vi "Read RFFE_w_Waveform.vi"(0 "Semiconductor Module Context":T3, 1 "USID":T1 max=15, 2 "Specific Bits Value_to_Read":cluster{"#ofBits":u8, "Bit_Location(LSB)":u8}={"#ofBits"=1, "Bit_Location(LSB)"=0} {"Bit_Location(LSB)" max=7; "#ofBits" min=1 max=8}, 5 "Pins":string[](array[string])=["CLK", "SDA"], 7 "RegisterAdd_Value_Dec":u8=28, 9 "Num_Reg_to_Read":u8, 11 "error in (no error)":errorcluster) -> (4 "Ext_Read_Reg":i32[](array[numeric]), 6 "Ext_Read_Data":u8[](array[numeric])=[31, 144, 7], 8 "Specific_Bits_Value":u8=184, 15 "error out":errorcluster)   [LabVIEW 2013]
uses:
  <vilib>/NI_TestStand_SemiconductorModule/NI_TestStand_Semiconductor_Module.lvlibp/PinMap/General/SemiconductorModuleContext.ctl
  Controls/USID.ctl
  MIPI_RFFE/Ctrls/RegReadWrite.ctl
  MIPI_RFFE/Ctrls/Configuration.ctl
  MIPI_RFFE/Ctrls/ClockDataChannels.ctl
  <instrlib>/niHSDIO/niHSDIO.llb/niHSDIO_ctl Generation Mode Values (Ring).ctl
  <vilib>/NI_TestStand_SemiconductorModule/NI_TestStand_Semiconductor_Module.lvlibp/PinMap/HSDIO/PinsToNIHSDIOSessions.vi
  <vilib>/Waveform/DWDTOps.llb/DWDT Digital Size.vi
  <instrlib>/niHSDIO/niHSDIO.llb/niHSDIO Write Named Waveform (WDT).vi
  <instrlib>/niHSDIO/niHSDIO.llb/niHSDIO Fetch Waveform (WDT).vi
  <vilib>/NI_TestStand_SemiconductorModule/NI_TestStand_Semiconductor_Module.lvlibp
panel:
  out "Converted Data":T2 {"Register" max=31 format="%.0x"; "Slave Address" max=15 format="%.0x"}
  out "Waveform Graph":digitalwaveform(graph)
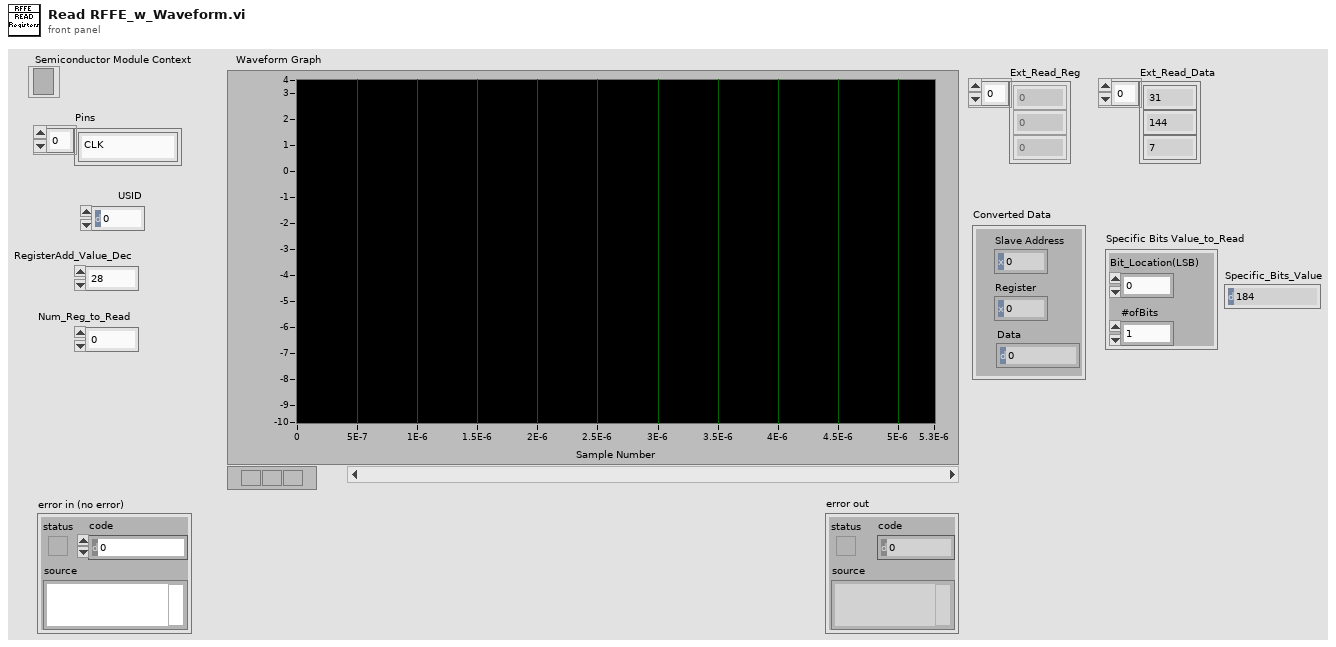
[diagram p1: front panel]
types:
  T1 = typedef "USID.ctl" = u8
  T2 = cluster{"Slave Address":u8, "Register":u8, "Data":u8}
  T3 = typedef "NI_TestStand_Semiconductor_Module.lvlibp/SemiconductorModuleContext.ctl" = refnum<k7>
  T4 = typedef "Configuration.ctl" = cluster{"Samples to Allocate":i32, "Oversample Factor":u8, "Clock Channel":T5, "Data Channel":T5}
  T5 = typedef "ClockDataChannels.ctl" = enum16{"0", "1"}
  T6 = typedef "RegReadWrite.ctl" = cluster{"Slave Address":u8, "Register":u8, "Data":u8, "SetID_Pin_State":enum16{"0", "1", "Z"}}
  T7 = typedef "niHSDIO_ctl Generation Mode Values (Ring).ctl" = i32
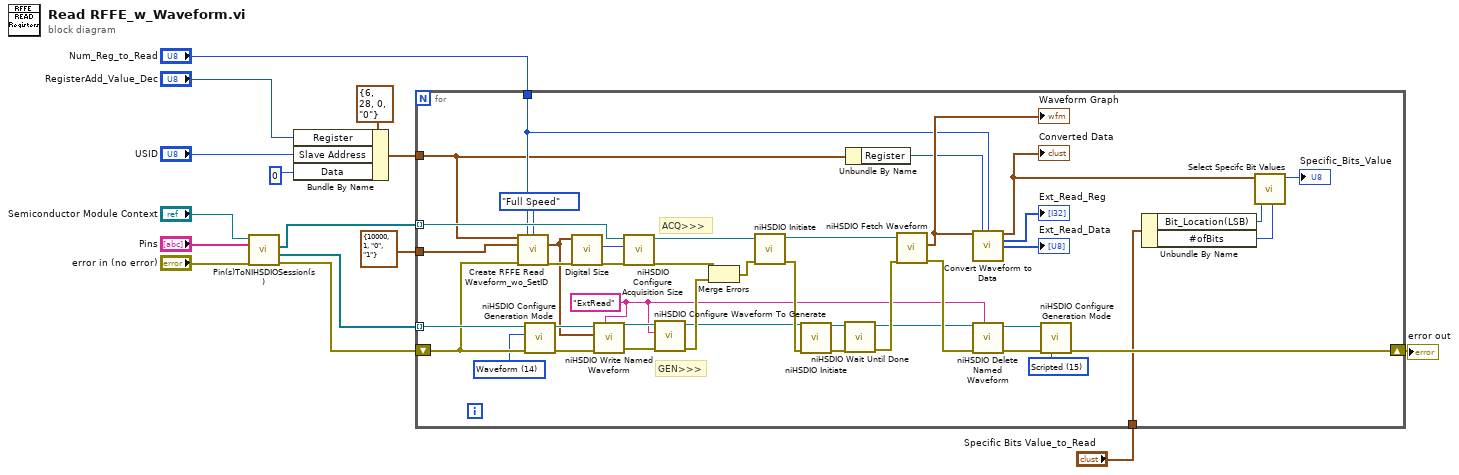
[diagram p0: block diagram]
diagram:
  n1 = call-poly <vilib>:"Pin(s)ToNIHSDIOSession(s).vi"("error in (no error)"="error in (no error)", "Pins"="Pins", "Semiconductor Module Context"="Semiconductor Module Context") -> ("error out"=w13:errorcluster, "Generation Sessions"=w14:refnum<k15>[], "Acquisition Sessions"=w15:refnum<k15>[])  [unwired: 3 in, 3 out]
  n2 = Bundle By Name(cluster=T6 {"Slave Address"=6, "Register"=28, "Data"=0, "SetID_Pin_State"=enum."0"} ("Data"), "Register"="RegisterAdd_Value_Dec", "Slave Address"="USID", "Data"=u8 0) -> (w8:T6)
  n3 = for {
    tunnel: w15 -> [w50] mode=indexing
    tunnel: w14 -> [w43] mode=indexing
    tunnel: w8 -> [w22]
    tunnel: T4 {"Samples to Allocate"=10000, "Oversample Factor"=1, "Clock Channel"=enum."0", "Data Channel"=enum."1"} ("Configuratation") -> [w48]
    shift-right: [w23] -> w6
    shift-left: w13 -> [w40]
    tunnel: "Num_Reg_to_Read" -> [w24]
    tunnel: "Specific Bits Value_to_Read" -> [w19]
    w34 = T7 15 items=["Waveform"=14, "Scripted"=15] ("generation mode (waveform)")
    w29 = "ExtRead" ("waveform name (default:\"\")")
    w39 = T7 14 items=["Waveform"=14, "Scripted"=15] ("generation mode (waveform)")
    # "GEN>>>"
    # "ACQ>>>"
    n4 = call "Create RFFE Read Waveform_wo_SetID.vi"("Data"=w22, "Ext_Read_Num_Reg"=w24, "Readback Speed"=enum16{"Full Speed", "Half Speed"}."Full Speed", "Configuratation"=w48, "error in (no error)"=w40) -> ("Waveform Graph"=w27:digitalwaveform, "error out"=w51:errorcluster)  [unwired: 9 in]
    n5 = call <instrlib>:"niHSDIO Configure Generation Mode.vi"("error in (no error)"=w40, "generation mode (waveform)"=w39, "instrument handle"=w43) -> ("error out"=w41:errorcluster, "instrument handle out"=w42:refnum<k15>)  [unwired: 7 in]
    n6 = call-poly <vilib>:"Digital Size.vi"("error in (no error)"=w51, "digital waveform in"=w27) -> ("error out"=w52:errorcluster, "number of samples"=w53:i32)  [unwired: 6 in, 2 out]
    n7 = call-poly <instrlib>:"niHSDIO Write Named Waveform.vi"("waveform name (default:\"\")"=w29, "error in (no error)"=w41, "data"=w27, "instrument handle"=w42) -> ("error out"=w38:errorcluster, "instrument handle out"=w36:refnum<k15>)  [unwired: 6 in]
    n8 = call <instrlib>:"niHSDIO Configure Acquisition Size.vi"("error in (no error)"=w52, "samples per record (1000 samples)"=w53, "instrument handle"=w50) -> ("error out"=w49:errorcluster, "instrument handle out"=w54:refnum<k15>)  [unwired: 7 in]
    n9 = call <instrlib>:"niHSDIO Configure Waveform To Generate.vi"("error in (no error)"=w38, "waveform name"=w29, "instrument handle"=w36) -> ("error out"=w37:errorcluster, "instrument handle out"=w35:refnum<k15>)  [unwired: 7 in]
    n10 = Merge Errors(w49, w37) -> (w55:errorcluster)
    n11 = call <instrlib>:"niHSDIO Initiate.vi"("error in (no error)"=w55, "instrument handle"=w54) -> ("error out"=w57:errorcluster, "instrument handle out"=w44:refnum<k15>)  [unwired: 8 in]
    n12 = call <instrlib>:"niHSDIO Initiate.vi"("error in (no error)"=w57, "instrument handle"=w35) -> ("error out"=w56:errorcluster, "instrument handle out"=w45:refnum<k15>)  [unwired: 8 in]
    n13 = call <instrlib>:"niHSDIO Wait Until Done.vi"("error in (no error)"=w56, "instrument handle"=w45) -> ("error out"=w47:errorcluster, "instrument handle out"=w31:refnum<k15>)  [unwired: 8 in]
    n14 = Unbundle By Name(w22) -> ("Register"=w21:u8)
    n15 = call-poly <instrlib>:"niHSDIO Fetch Waveform.vi"("error in (no error)"=w47, "instrument handle"=w44) -> ("error out"=w33:errorcluster, "data"=w28:digitalwaveform)  [unwired: 6 in, 2 out]
    "Waveform Graph" <- w28
    n16 = call "Convert Waveform to Data.vi"("Waveform Graph"=w28, "Register"=w21, "Ext_Read_Num_Reg"=w24) -> ("Converted Data"=w20:T2, "Ext_Read_Reg"=→"Ext_Read_Reg":i32[], "Ext_Read_Data"=→"Ext_Read_Data":u8[])  [unwired: 10 in]
    "Converted Data" <- w20
    n17 = call <instrlib>:"niHSDIO Delete Named Waveform.vi"("waveform name (default:\"\")"=w29, "error in (no error)"=w33, "instrument handle"=w31) -> ("error out"=w32:errorcluster, "instrument handle out"=w30:refnum<k15>)  [unwired: 7 in]
    n18 = call <instrlib>:"niHSDIO Configure Generation Mode.vi"("error in (no error)"=w32, "generation mode (waveform)"=w34, "instrument handle"=w30) -> ("error out"=w23:errorcluster)  [unwired: 7 in, 1 out]
    n19 = Unbundle By Name(w19) -> ("Bit_Location(LSB)"=w18:u8, "#ofBits"=w17:u8)
    n20 = call "Select Specifc Bit Values.vi"("#ofBits"=w17, "Bit_Location(LSB)"=w18, "Converted Data"=w20) -> ("Bits"=→"Specific_Bits_Value":u8)  [unwired: 8 in]
  }
  "error out" <- w6
